vi "Read EDS File.vi"(8 "error in":errorcluster, 10 "EDS File Path":path, 11 "UI Actor in":refnum<class "UI Actor.lvclass">) -> (0 "error out":errorcluster, 3 "UI Actor out":refnum<class "UI Actor.lvclass">)   [LabVIEW 2024, in "UI Actor.lvlib" / "UI Actor.lvclass"]
uses:
  UI Actor.lvclass
  UI Actor.lvclass/UI Actor.ctl
  Electronic Datasheet/Electronic Datasheet.lvclass
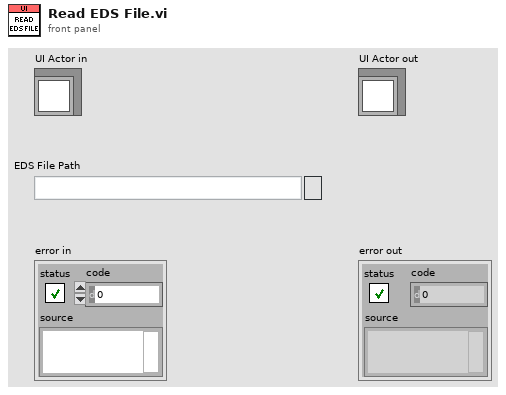
[diagram p1: front panel]
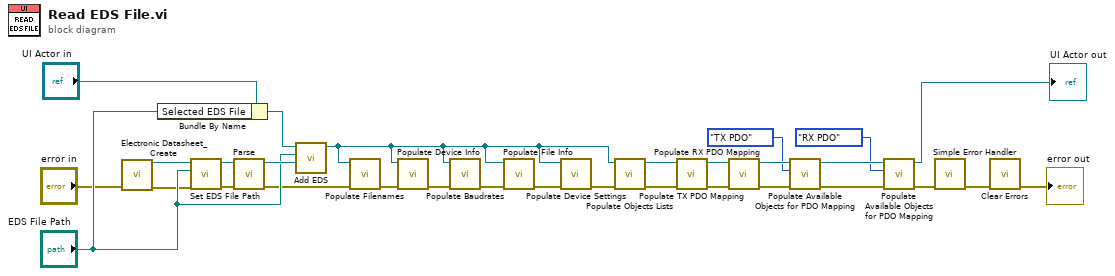
[diagram p0: block diagram]
diagram:
  n1 = call "Electronic Datasheet_Create.vi"("Error In"="error in") -> ("Error Out"=w21:errorcluster, "reference out"=w22:refnum<class "Electronic Datasheet.lvclass">)  [unwired: 9 in]
  n2 = Bundle By Name(cluster="UI Actor in", "Selected EDS File"="EDS File Path") -> (w27:refnum<class "UI Actor.lvclass">)
  n3 = call "Set EDS File Path.vi"("error in"=w21, "EDS File Path"="EDS File Path", "reference in"=w22) -> ("error out"=w20:errorcluster, "reference out"=w30:refnum<class "Electronic Datasheet.lvclass">)  [unwired: 7 in]
  n4 = call "Parse.vi"("error in"=w20, "reference in"=w30) -> ("error out"=w25:errorcluster, "reference out"=w29:refnum<class "Electronic Datasheet.lvclass">)  [unwired: 8 in]
  n5 = call "Add EDS.vi"("EDS"=w29, "File Path"="EDS File Path", "UI Actor in"=w27) -> ("UI Actor out"=w6:refnum<class "UI Actor.lvclass">)  [unwired: 8 in]
  n6 = call "Populate Filenames.vi"("error in"=w25, "UI Actor in"=w6) -> ("error out"=w19:errorcluster)  [unwired: 9 in]
  n7 = call "Populate Device Info.vi"("error in"=w19, "UI Actor in"=w6) -> ("error out"=w11:errorcluster)  [unwired: 9 in]
  n8 = call "Populate Baudrates.vi"("error in"=w11, "UI Actor in"=w6) -> ("error out"=w12:errorcluster)  [unwired: 9 in]
  n9 = call "Populate File Info.vi"("error in"=w12, "UI Actor in"=w6) -> ("error out"=w13:errorcluster)  [unwired: 9 in]
  n10 = call "Populate Device Settings.vi"("error in"=w13, "UI Actor in"=w6) -> ("error out"=w14:errorcluster)  [unwired: 9 in]
  n11 = call "Populate Objects Lists.vi"("error in"=w14, "UI Actor in"=w6) -> ("error out"=w15:errorcluster, "UI Actor out"=w7:refnum<class "UI Actor.lvclass">)  [unwired: 8 in]
  n12 = call "Populate TX PDO Mapping.vi"("error in"=w15, "UI Actor in"=w7) -> ("error out"=w16:errorcluster, "UI Actor out"=w10:refnum<class "UI Actor.lvclass">)  [unwired: 8 in]
  n13 = call "Populate RX PDO Mapping.vi"("error in"=w16, "UI Actor in"=w10) -> ("error out"=w17:errorcluster, "UI Actor out"=w8:refnum<class "UI Actor.lvclass">)  [unwired: 8 in]
  n14 = call "Populate Available Objects for PDO Mapping.vi"("error in"=w17, "Type"=enum16{"TX PDO", "RX PDO"}."TX PDO", "UI Actor in"=w8) -> ("error out"=w9:errorcluster, "UI Actor out"=w3:refnum<class "UI Actor.lvclass">)  [unwired: 7 in]
  n15 = call "Populate Available Objects for PDO Mapping.vi"("error in"=w9, "Type"=enum16{"TX PDO", "RX PDO"}."RX PDO", "UI Actor in"=w3) -> ("error out"=w4:errorcluster, "UI Actor out"=→"UI Actor out":refnum<class "UI Actor.lvclass">)  [unwired: 7 in]
  n16 = call <vilib>:"Simple Error Handler.vi"("error in (no error)"=w4) -> ("error out"=w24:errorcluster)  [unwired: 4 in, 4 out]
  n17 = call <vilib>:"Clear Errors.vi"("error in (no error)"=w24) -> ("error out"=→"error out":errorcluster)  [unwired: 5 in, 1 out]
